vi "Lab Panel V5.24.vi"() -> ()   [LabVIEW 2013] (continued)
                      tunnel: w2146 -> [w2161 _]
                      tunnel: w2145 -> [w2160 _]
                      tunnel: w2144 -> [w2159 _]
                      frame True {
                        n1125 = stacked-sequence {
                          tunnel: w2162 -> [w2166 _]
                          tunnel: w2161 -> [w2164 w2170]
                          tunnel: w2160 -> [_ w2173]
                          tunnel: w2159 -> [w2163 _]
                          frame #0 {
                            n1126 = Build Array(w2164) -> (w2167:string[])
                            n1127 = Build Array(w2166) -> (w2165:dbl[])
                            n1128 = TDMS Write(0:w2163, 5:"TEST PASS", 7:w2167, 9:w2165) -> (15:w2169:errorcluster)  [unwired: 2 in, 3 out]
                            n1129 = local write "data file error"(w2169) -> ()
                          }
                          frame #1 {
                            n1130 = Bundle(cluster=w2173, "STATUS"=w2170) -> (w2171:T4)  [unwired: 2 in]
                            n1131 = local write "RESULT LAB01-2"(TRUE) -> ()
                            n1132 = local write "DISP LAB01-2"(w2171) -> ()
                          }
                        }
                      }
                      frame False {
                      }
                    }
                  }
                }
              }
              frame #2 {
                # "LAB02-1"
                n1133 = Less?(x=w2174, y=2) -> (x < y?=w2177:bool)
                n1134 = local read "DISP LAB02-1"() -> (w2179:T4)
                n1135 = Unbundle(w2179) -> ("STATUS"=w2180:string)  [unwired: 2 out]
                n1136 = Equal?(x=w2180, y="RUN") -> (x = y?=w2176:bool)
                n1137 = And(x=w2176, y=w2177) -> (x .and. y?=w2175:bool)
                n1138 = case shown="True" w2175 {
                  tunnel: w2179 -> [_ w2185]
                  tunnel: w2174 -> [_ w2189]
                  frame False {
                  }
                  frame True {
                    n1139 = local read "SET LAB02-1"() -> (w2191:T5)
                    n1140 = local read "TDMS LAB02-1"() -> (w2184:refnum<k34>)
                    n1141 = Unbundle(w2185) -> ("CYCLE"=w2190:dbl)  [unwired: 2 out]
                    n1142 = Unbundle(w2191) -> ("CYCLES"=w2182:dbl, "T-RISE mins"=w2188:dbl)  [unwired: 3 out]
                    n1143 = case shown="\"T-RISE TEST\"" w2189 {
                      tunnel: w2188 -> [_ _ w2198]
                      tunnel: [w2193 w2195 w2198] -> w2187
                      tunnel: w2182 -> [w2193 w2195 _]
                      tunnel: ["CHART PASS" "CYCLE PASS" "T-RISE PASS"] -> w2186
                      frame "CHART TEST", Default {
                      }
                      frame "CYCLE TEST" {
                      }
                      frame "T-RISE TEST" {
                      }
                    }
                    n1144 = Increment(x=w2182) -> (x+1=w2183:dbl)
                    n1145 = Greater Or Equal?(x=w2190, y=w2183) -> (x >= y?=w2192:bool)
                    n1146 = case shown="True" w2192 {
                      tunnel: w2187 -> [w2202 _]
                      tunnel: w2186 -> [w2201 _]
                      tunnel: w2185 -> [w2200 _]
                      tunnel: w2184 -> [w2199 _]
                      frame True {
                        n1147 = stacked-sequence {
                          tunnel: w2202 -> [w2206 _]
                          tunnel: w2201 -> [w2204 w2210]
                          tunnel: w2200 -> [_ w2213]
                          tunnel: w2199 -> [w2203 _]
                          frame #0 {
                            n1148 = Build Array(w2204) -> (w2207:string[])
                            n1149 = Build Array(w2206) -> (w2205:dbl[])
                            n1150 = TDMS Write(0:w2203, 5:"TEST PASS", 7:w2207, 9:w2205) -> (15:w2209:errorcluster)  [unwired: 2 in, 3 out]
                            n1151 = local write "data file error"(w2209) -> ()
                          }
                          frame #1 {
                            n1152 = Bundle(cluster=w2213, "STATUS"=w2210) -> (w2211:T4)  [unwired: 2 in]
                            n1153 = local write "RESULT LAB02-1"(TRUE) -> ()
                            n1154 = local write "DISP LAB02-1"(w2211) -> ()
                          }
                        }
                      }
                      frame False {
                      }
                    }
                  }
                }
              }
              frame #3 {
                # "LAB02-2"
                n1155 = Less?(x=w2214, y=2) -> (x < y?=w2217:bool)
                n1156 = local read "DISP LAB02-2"() -> (w2219:T4)
                n1157 = Unbundle(w2219) -> ("STATUS"=w2220:string)  [unwired: 2 out]
                n1158 = Equal?(x=w2220, y="RUN") -> (x = y?=w2216:bool)
                n1159 = And(x=w2216, y=w2217) -> (x .and. y?=w2215:bool)
                n1160 = case shown="True" w2215 {
                  tunnel: w2219 -> [_ w2225]
                  tunnel: w2214 -> [_ w2229]
                  frame False {
                  }
                  frame True {
                    n1161 = local read "SET LAB02-2"() -> (w2231:T5)
                    n1162 = local read "TDMS LAB02-2"() -> (w2224:refnum<k34>)
                    n1163 = Unbundle(w2225) -> ("CYCLE"=w2230:dbl)  [unwired: 2 out]
                    n1164 = Unbundle(w2231) -> ("CYCLES"=w2222:dbl, "T-RISE mins"=w2228:dbl)  [unwired: 3 out]
                    n1165 = case shown="\"T-RISE TEST\"" w2229 {
                      tunnel: w2228 -> [_ _ w2238]
                      tunnel: [w2233 w2235 w2238] -> w2227
                      tunnel: w2222 -> [w2233 w2235 _]
                      tunnel: ["CHART PASS" "CYCLE PASS" "T-RISE PASS"] -> w2226
                      frame "CHART TEST", Default {
                      }
                      frame "CYCLE TEST" {
                      }
                      frame "T-RISE TEST" {
                      }
                    }
                    n1166 = Increment(x=w2222) -> (x+1=w2223:dbl)
                    n1167 = Greater Or Equal?(x=w2230, y=w2223) -> (x >= y?=w2232:bool)
                    n1168 = case shown="True" w2232 {
                      tunnel: w2227 -> [w2242 _]
                      tunnel: w2226 -> [w2241 _]
                      tunnel: w2225 -> [w2240 _]
                      tunnel: w2224 -> [w2239 _]
                      frame True {
                        n1169 = stacked-sequence {
                          tunnel: w2242 -> [w2246 _]
                          tunnel: w2241 -> [w2244 w2250]
                          tunnel: w2240 -> [_ w2253]
                          tunnel: w2239 -> [w2243 _]
                          frame #0 {
                            n1170 = Build Array(w2244) -> (w2247:string[])
                            n1171 = Build Array(w2246) -> (w2245:dbl[])
                            n1172 = TDMS Write(0:w2243, 5:"TEST PASS", 7:w2247, 9:w2245) -> (15:w2249:errorcluster)  [unwired: 2 in, 3 out]
                            n1173 = local write "data file error"(w2249) -> ()
                          }
                          frame #1 {
                            n1174 = Bundle(cluster=w2253, "STATUS"=w2250) -> (w2251:T4)  [unwired: 2 in]
                            n1175 = local write "RESULT LAB02-2"(TRUE) -> ()
                            n1176 = local write "DISP LAB02-2"(w2251) -> ()
                          }
                        }
                      }
                      frame False {
                      }
                    }
                  }
                }
              }
              frame #4 {
                # "LAB03-1"
                n1177 = Less?(x=w2254, y=2) -> (x < y?=w2257:bool)
                n1178 = local read "DISP LAB03-1"() -> (w2259:T4)
                n1179 = Unbundle(w2259) -> ("STATUS"=w2260:string)  [unwired: 2 out]
                n1180 = Equal?(x=w2260, y="RUN") -> (x = y?=w2256:bool)
                n1181 = And(x=w2256, y=w2257) -> (x .and. y?=w2255:bool)
                n1182 = case shown="True" w2255 {
                  tunnel: w2259 -> [_ w2265]
                  tunnel: w2254 -> [_ w2269]
                  frame False {
                  }
                  frame True {
                    n1183 = local read "SET LAB03-1"() -> (w2271:T5)
                    n1184 = local read "TDMS LAB03-1"() -> (w2264:refnum<k34>)
                    n1185 = Unbundle(w2265) -> ("CYCLE"=w2270:dbl)  [unwired: 2 out]
                    n1186 = Unbundle(w2271) -> ("CYCLES"=w2262:dbl, "T-RISE mins"=w2268:dbl)  [unwired: 3 out]
                    n1187 = case shown="\"T-RISE TEST\"" w2269 {
                      tunnel: w2268 -> [_ _ w2278]
                      tunnel: [w2273 w2275 w2278] -> w2267
                      tunnel: w2262 -> [w2273 w2275 _]
                      tunnel: ["CHART PASS" "CYCLE PASS" "T-RISE PASS"] -> w2266
                      frame "CHART TEST", Default {
                      }
                      frame "CYCLE TEST" {
                      }
                      frame "T-RISE TEST" {
                      }
                    }
                    n1188 = Increment(x=w2262) -> (x+1=w2263:dbl)
                    n1189 = Greater Or Equal?(x=w2270, y=w2263) -> (x >= y?=w2272:bool)
                    n1190 = case shown="True" w2272 {
                      tunnel: w2267 -> [w2282 _]
                      tunnel: w2266 -> [w2281 _]
                      tunnel: w2265 -> [w2280 _]
                      tunnel: w2264 -> [w2279 _]
                      frame True {
                        n1191 = stacked-sequence {
                          tunnel: w2282 -> [w2286 _]
                          tunnel: w2281 -> [w2284 w2290]
                          tunnel: w2280 -> [_ w2293]
                          tunnel: w2279 -> [w2283 _]
                          frame #0 {
                            n1192 = Build Array(w2284) -> (w2287:string[])
                            n1193 = Build Array(w2286) -> (w2285:dbl[])
                            n1194 = TDMS Write(0:w2283, 5:"TEST PASS", 7:w2287, 9:w2285) -> (15:w2289:errorcluster)  [unwired: 2 in, 3 out]
                            n1195 = local write "data file error"(w2289) -> ()
                          }
                          frame #1 {
                            n1196 = Bundle(cluster=w2293, "STATUS"=w2290) -> (w2291:T4)  [unwired: 2 in]
                            n1197 = local write "RESULT LAB03-1"(TRUE) -> ()
                            n1198 = local write "DISP LAB03-1"(w2291) -> ()
                          }
                        }
                      }
                      frame False {
                      }
                    }
                  }
                }
              }
              frame #5 {
                # "LAB03-2"
                n1199 = Less?(x=w2294, y=2) -> (x < y?=w2297:bool)
                n1200 = local read "DISP LAB03-2"() -> (w2299:T4)
                n1201 = Unbundle(w2299) -> ("STATUS"=w2300:string)  [unwired: 2 out]
                n1202 = Equal?(x=w2300, y="RUN") -> (x = y?=w2296:bool)
                n1203 = And(x=w2296, y=w2297) -> (x .and. y?=w2295:bool)
                n1204 = case shown="True" w2295 {
                  tunnel: w2299 -> [_ w2305]
                  tunnel: w2294 -> [_ w2309]
                  frame False {
                  }
                  frame True {
                    n1205 = local read "SET LAB03-2"() -> (w2311:T5)
                    n1206 = local read "TDMS LAB03-2"() -> (w2304:refnum<k34>)
                    n1207 = Unbundle(w2305) -> ("CYCLE"=w2310:dbl)  [unwired: 2 out]
                    n1208 = Unbundle(w2311) -> ("CYCLES"=w2302:dbl, "T-RISE mins"=w2308:dbl)  [unwired: 3 out]
                    n1209 = case shown="\"T-RISE TEST\"" w2309 {
                      tunnel: w2308 -> [_ _ w2318]
                      tunnel: [w2313 w2315 w2318] -> w2307
                      tunnel: w2302 -> [w2313 w2315 _]
                      tunnel: ["CHART PASS" "CYCLE PASS" "T-RISE PASS"] -> w2306
                      frame "CHART TEST", Default {
                      }
                      frame "CYCLE TEST" {
                      }
                      frame "T-RISE TEST" {
                      }
                    }
                    n1210 = Increment(x=w2302) -> (x+1=w2303:dbl)
                    n1211 = Greater Or Equal?(x=w2310, y=w2303) -> (x >= y?=w2312:bool)
                    n1212 = case shown="True" w2312 {
                      tunnel: w2307 -> [w2322 _]
                      tunnel: w2306 -> [w2321 _]
                      tunnel: w2305 -> [w2320 _]
                      tunnel: w2304 -> [w2319 _]
                      frame True {
                        n1213 = stacked-sequence {
                          tunnel: w2322 -> [w2326 _]
                          tunnel: w2321 -> [w2324 w2330]
                          tunnel: w2320 -> [_ w2333]
                          tunnel: w2319 -> [w2323 _]
                          frame #0 {
                            n1214 = Build Array(w2324) -> (w2327:string[])
                            n1215 = Build Array(w2326) -> (w2325:dbl[])
                            n1216 = TDMS Write(0:w2323, 5:"TEST PASS", 7:w2327, 9:w2325) -> (15:w2329:errorcluster)  [unwired: 2 in, 3 out]
                            n1217 = local write "data file error"(w2329) -> ()
                          }
                          frame #1 {
                            n1218 = Bundle(cluster=w2333, "STATUS"=w2330) -> (w2331:T4)  [unwired: 2 in]
                            n1219 = local write "RESULT LAB03-2"(TRUE) -> ()
                            n1220 = local write "DISP LAB03-2"(w2331) -> ()
                          }
                        }
                      }
                      frame False {
                      }
                    }
                  }
                }
              }
              frame #6 {
                # "LAB04-1"
                n1221 = Less?(x=w2334, y=2) -> (x < y?=w2337:bool)
                n1222 = local read "DISP LAB04-1"() -> (w2339:T4)
                n1223 = Unbundle(w2339) -> ("STATUS"=w2340:string)  [unwired: 2 out]
                n1224 = Equal?(x=w2340, y="RUN") -> (x = y?=w2336:bool)
                n1225 = And(x=w2336, y=w2337) -> (x .and. y?=w2335:bool)
                n1226 = case shown="True" w2335 {
                  tunnel: w2339 -> [_ w2345]
                  tunnel: w2334 -> [_ w2349]
                  frame False {
                  }
                  frame True {
                    n1227 = local read "SET LAB04-1"() -> (w2351:T5)
                    n1228 = local read "TDMS LAB04-1"() -> (w2344:refnum<k34>)
                    n1229 = Unbundle(w2345) -> ("CYCLE"=w2350:dbl)  [unwired: 2 out]
                    n1230 = Unbundle(w2351) -> ("CYCLES"=w2342:dbl, "T-RISE mins"=w2348:dbl)  [unwired: 3 out]
                    n1231 = case shown="\"T-RISE TEST\"" w2349 {
                      tunnel: w2348 -> [_ _ w2358]
                      tunnel: [w2353 w2355 w2358] -> w2347
                      tunnel: w2342 -> [w2353 w2355 _]
                      tunnel: ["CHART PASS" "CYCLE PASS" "T-RISE PASS"] -> w2346
                      frame "CHART TEST", Default {
                      }
                      frame "CYCLE TEST" {
                      }
                      frame "T-RISE TEST" {
                      }
                    }
                    n1232 = Increment(x=w2342) -> (x+1=w2343:dbl)
                    n1233 = Greater Or Equal?(x=w2350, y=w2343) -> (x >= y?=w2352:bool)
                    n1234 = case shown="True" w2352 {
                      tunnel: w2347 -> [w2362 _]
                      tunnel: w2346 -> [w2361 _]
                      tunnel: w2345 -> [w2360 _]
                      tunnel: w2344 -> [w2359 _]
                      frame True {
                        n1235 = stacked-sequence {
                          tunnel: w2362 -> [w2366 _]
                          tunnel: w2361 -> [w2364 w2370]
                          tunnel: w2360 -> [_ w2373]
                          tunnel: w2359 -> [w2363 _]
                          frame #0 {
                            n1236 = Build Array(w2364) -> (w2367:string[])
                            n1237 = Build Array(w2366) -> (w2365:dbl[])
                            n1238 = TDMS Write(0:w2363, 5:"TEST PASS", 7:w2367, 9:w2365) -> (15:w2369:errorcluster)  [unwired: 2 in, 3 out]
                            n1239 = local write "data file error"(w2369) -> ()
                          }
                          frame #1 {
                            n1240 = Bundle(cluster=w2373, "STATUS"=w2370) -> (w2371:T4)  [unwired: 2 in]
                            n1241 = local write "RESULT LAB04-1"(TRUE) -> ()
                            n1242 = local write "DISP LAB04-1"(w2371) -> ()
                          }
                        }
                      }
                      frame False {
                      }
                    }
                  }
                }
              }
              frame #7 {
                # "LAB04-2"
                n1243 = Less?(x=w2374, y=2) -> (x < y?=w2377:bool)
                n1244 = local read "DISP LAB04-2"() -> (w2379:T4)
                n1245 = Unbundle(w2379) -> ("STATUS"=w2380:string)  [unwired: 2 out]
                n1246 = Equal?(x=w2380, y="RUN") -> (x = y?=w2376:bool)
                n1247 = And(x=w2376, y=w2377) -> (x .and. y?=w2375:bool)
                n1248 = case shown="True" w2375 {
                  tunnel: w2379 -> [_ w2385]
                  tunnel: w2374 -> [_ w2389]
                  frame False {
                  }
                  frame True {
                    n1249 = local read "SET LAB04-2"() -> (w2391:T5)
                    n1250 = local read "TDMS LAB04-2"() -> (w2384:refnum<k34>)
                    n1251 = Unbundle(w2385) -> ("CYCLE"=w2390:dbl)  [unwired: 2 out]
                    n1252 = Unbundle(w2391) -> ("CYCLES"=w2382:dbl, "T-RISE mins"=w2388:dbl)  [unwired: 3 out]
                    n1253 = case shown="\"T-RISE TEST\"" w2389 {
                      tunnel: w2388 -> [_ _ w2398]
                      tunnel: [w2393 w2395 w2398] -> w2387
                      tunnel: w2382 -> [w2393 w2395 _]
                      tunnel: ["CHART PASS" "CYCLE PASS" "T-RISE PASS"] -> w2386
                      frame "CHART TEST", Default {
                      }
                      frame "CYCLE TEST" {
                      }
                      frame "T-RISE TEST" {
                      }
                    }
                    n1254 = Increment(x=w2382) -> (x+1=w2383:dbl)
                    n1255 = Greater Or Equal?(x=w2390, y=w2383) -> (x >= y?=w2392:bool)
                    n1256 = case shown="True" w2392 {
                      tunnel: w2387 -> [w2402 _]
                      tunnel: w2386 -> [w2401 _]
                      tunnel: w2385 -> [w2400 _]
                      tunnel: w2384 -> [w2399 _]
                      frame True {
                        n1257 = stacked-sequence {
                          tunnel: w2402 -> [w2406 _]
                          tunnel: w2401 -> [w2404 w2410]
                          tunnel: w2400 -> [_ w2413]
                          tunnel: w2399 -> [w2403 _]
                          frame #0 {
                            n1258 = Build Array(w2404) -> (w2407:string[])
                            n1259 = Build Array(w2406) -> (w2405:dbl[])
                            n1260 = TDMS Write(0:w2403, 5:"TEST PASS", 7:w2407, 9:w2405) -> (15:w2409:errorcluster)  [unwired: 2 in, 3 out]
                            n1261 = local write "data file error"(w2409) -> ()
                          }
                          frame #1 {
                            n1262 = Bundle(cluster=w2413, "STATUS"=w2410) -> (w2411:T4)  [unwired: 2 in]
                            n1263 = local write "RESULT LAB04-2"(TRUE) -> ()
                            n1264 = local write "DISP LAB04-2"(w2411) -> ()
                          }
                        }
                      }
                      frame False {
                      }
                    }
                  }
                }
              }
              frame #8 {
                # "LAB05-1"
                n1265 = Less?(x=w2414, y=2) -> (x < y?=w2417:bool)
                n1266 = local read "DISP LAB05-1"() -> (w2419:T4)
                n1267 = Unbundle(w2419) -> ("STATUS"=w2420:string)  [unwired: 2 out]
                n1268 = Equal?(x=w2420, y="RUN") -> (x = y?=w2416:bool)
                n1269 = And(x=w2416, y=w2417) -> (x .and. y?=w2415:bool)
                n1270 = case shown="True" w2415 {
                  tunnel: w2419 -> [_ w2425]
                  tunnel: w2414 -> [_ w2429]
                  frame False {
                  }
                  frame True {
                    n1271 = local read "SET LAB05-1"() -> (w2431:T5)
                    n1272 = local read "TDMS LAB05-1"() -> (w2424:refnum<k34>)
                    n1273 = Unbundle(w2425) -> ("CYCLE"=w2430:dbl)  [unwired: 2 out]
                    n1274 = Unbundle(w2431) -> ("CYCLES"=w2422:dbl, "T-RISE mins"=w2428:dbl)  [unwired: 3 out]
                    n1275 = case shown="\"T-RISE TEST\"" w2429 {
                      tunnel: w2428 -> [_ _ w2438]
                      tunnel: [w2433 w2435 w2438] -> w2427
                      tunnel: w2422 -> [w2433 w2435 _]
                      tunnel: ["CHART PASS" "CYCLE PASS" "T-RISE PASS"] -> w2426
                      frame "CHART TEST", Default {
                      }
                      frame "CYCLE TEST" {
                      }
                      frame "T-RISE TEST" {
                      }
                    }
                    n1276 = Increment(x=w2422) -> (x+1=w2423:dbl)
                    n1277 = Greater Or Equal?(x=w2430, y=w2423) -> (x >= y?=w2432:bool)
                    n1278 = case shown="True" w2432 {
                      tunnel: w2427 -> [w2442 _]
                      tunnel: w2426 -> [w2441 _]
                      tunnel: w2425 -> [w2440 _]
                      tunnel: w2424 -> [w2439 _]
                      frame True {
                        n1279 = stacked-sequence {
                          tunnel: w2442 -> [w2446 _]
                          tunnel: w2441 -> [w2444 w2450]
                          tunnel: w2440 -> [_ w2453]
                          tunnel: w2439 -> [w2443 _]
                          frame #0 {
                            n1280 = Build Array(w2444) -> (w2447:string[])
                            n1281 = Build Array(w2446) -> (w2445:dbl[])
                            n1282 = TDMS Write(0:w2443, 5:"TEST PASS", 7:w2447, 9:w2445) -> (15:w2449:errorcluster)  [unwired: 2 in, 3 out]
                            n1283 = local write "data file error"(w2449) -> ()
                          }
                          frame #1 {
                            n1284 = Bundle(cluster=w2453, "STATUS"=w2450) -> (w2451:T4)  [unwired: 2 in]
                            n1285 = local write "RESULT LAB05-1"(TRUE) -> ()
                            n1286 = local write "DISP LAB05-1"(w2451) -> ()
                          }
                        }
                      }
                      frame False {
                      }
                    }
                  }
                }
              }
              frame #9 {
                # "LAB05-2"
                n1287 = Less?(x=w2454, y=2) -> (x < y?=w2457:bool)
                n1288 = local read "DISP LAB05-2"() -> (w2459:T4)
                n1289 = Unbundle(w2459) -> ("STATUS"=w2460:string)  [unwired: 2 out]
                n1290 = Equal?(x=w2460, y="RUN") -> (x = y?=w2456:bool)
                n1291 = And(x=w2456, y=w2457) -> (x .and. y?=w2455:bool)
                n1292 = case shown="True" w2455 {
                  tunnel: w2459 -> [_ w2465]
                  tunnel: w2454 -> [_ w2469]
                  frame False {
                  }
                  frame True {
                    n1293 = local read "SET LAB05-2"() -> (w2471:T5)
                    n1294 = local read "TDMS LAB05-2"() -> (w2464:refnum<k34>)
                    n1295 = Unbundle(w2465) -> ("CYCLE"=w2470:dbl)  [unwired: 2 out]
                    n1296 = Unbundle(w2471) -> ("CYCLES"=w2462:dbl, "T-RISE mins"=w2468:dbl)  [unwired: 3 out]
                    n1297 = case shown="\"T-RISE TEST\"" w2469 {
                      tunnel: w2468 -> [_ _ w2478]
                      tunnel: [w2473 w2475 w2478] -> w2467
                      tunnel: w2462 -> [w2473 w2475 _]
                      tunnel: ["CHART PASS" "CYCLE PASS" "T-RISE PASS"] -> w2466
                      frame "CHART TEST", Default {
                      }
                      frame "CYCLE TEST" {
                      }
                      frame "T-RISE TEST" {
                      }
                    }
                    n1298 = Increment(x=w2462) -> (x+1=w2463:dbl)
                    n1299 = Greater Or Equal?(x=w2470, y=w2463) -> (x >= y?=w2472:bool)
                    n1300 = case shown="True" w2472 {
                      tunnel: w2467 -> [w2482 _]
                      tunnel: w2466 -> [w2481 _]
                      tunnel: w2465 -> [w2480 _]
                      tunnel: w2464 -> [w2479 _]
                      frame True {
                        n1301 = stacked-sequence {
                          tunnel: w2482 -> [w2486 _]
                          tunnel: w2481 -> [w2484 w2490]
                          tunnel: w2480 -> [_ w2493]
                          tunnel: w2479 -> [w2483 _]
                          frame #0 {
                            n1302 = Build Array(w2484) -> (w2487:string[])
                            n1303 = Build Array(w2486) -> (w2485:dbl[])
                            n1304 = TDMS Write(0:w2483, 5:"TEST PASS", 7:w2487, 9:w2485) -> (15:w2489:errorcluster)  [unwired: 2 in, 3 out]
                            n1305 = local write "data file error"(w2489) -> ()
                          }
                          frame #1 {
                            n1306 = Bundle(cluster=w2493, "STATUS"=w2490) -> (w2491:T4)  [unwired: 2 in]
                            n1307 = local write "RESULT LAB05-2"(TRUE) -> ()
                            n1308 = local write "DISP LAB05-2"(w2491) -> ()
                          }
                        }
                      }
                      frame False {
                      }
                    }
                  }
                }
              }
            }
          }
          frame #5 {
            # "check if test cycles reached for temperature rise test"
            n1309 = stacked-sequence {
              tunnel: w2523 -> [_ _ _ _ _ _ _ _ _ _]
              tunnel: w2522 -> [_ _ _ _ _ _ _ _ _ _]
              tunnel: w2521 -> [_ _ _ _ _ _ _ _ _ _]
              tunnel: w2520 -> [_ _ _ _ _ _ _ _ _ _]
              tunnel: w2519 -> [_ _ _ _ _ _ _ _ _ _]
              tunnel: w2518 -> [_ _ _ _ _ _ _ _ _ _]
              tunnel: w2517 -> [_ _ _ _ _ _ _ _ _ _]
              tunnel: w2516 -> [_ _ _ _ _ _ _ _ _ _]
              tunnel: w2515 -> [_ _ _ _ _ _ _ _ _ _]
              tunnel: w2514 -> [_ _ _ _ _ _ _ _ _ _]
              tunnel: w2513 -> [w2529 _ _ _ _ _ _ _ _ _]
              tunnel: w2503 -> [w2524 _ _ _ _ _ _ _ _ _]
              tunnel: w2512 -> [_ w2555 _ _ _ _ _ _ _ _]
              tunnel: w2511 -> [_ _ w2585 _ _ _ _ _ _ _]
              tunnel: w2510 -> [_ _ _ w2615 _ _ _ _ _ _]
              tunnel: w2509 -> [_ _ _ _ w2645 _ _ _ _ _]
              tunnel: w2508 -> [_ _ _ _ _ w2675 _ _ _ _]
              tunnel: w2507 -> [_ _ _ _ _ _ w2705 _ _ _]
              tunnel: w2506 -> [_ _ _ _ _ _ _ w2735 _ _]
              tunnel: w2505 -> [_ _ _ _ _ _ _ _ w2765 _]
              tunnel: w2504 -> [_ _ _ _ _ _ _ _ _ w2795]
              tunnel: w2502 -> [_ w2554 _ _ _ _ _ _ _ _]
              tunnel: w2501 -> [_ _ w2584 _ _ _ _ _ _ _]
              tunnel: w2500 -> [_ _ _ w2614 _ _ _ _ _ _]
              tunnel: w2499 -> [_ _ _ _ w2644 _ _ _ _ _]
              tunnel: w2498 -> [_ _ _ _ _ w2674 _ _ _ _]
              tunnel: w2497 -> [_ _ _ _ _ _ w2704 _ _ _]
              tunnel: w2496 -> [_ _ _ _ _ _ _ w2734 _ _]
              tunnel: w2495 -> [_ _ _ _ _ _ _ _ w2764 _]
              tunnel: w2494 -> [_ _ _ _ _ _ _ _ _ w2794]
              frame #0 {
                # "LAB01-1"
                n1310 = Equal?(x=w2529, y=2) -> (x = y?=w2527:bool)
                n1311 = local read "DISP LAB01-1"() -> (w2530:T4)
                n1312 = Unbundle(w2530) -> ("STATUS"=w2531:string)  [unwired: 2 out]
                n1313 = Equal?(x=w2531, y="RUN") -> (x = y?=w2526:bool)
                n1314 = And(x=w2526, y=w2527) -> (x .and. y?=w2525:bool)
                n1315 = case shown="True" w2525 {
                  tunnel: w2530 -> [_ w2534]
                  tunnel: w2524 -> [_ w2537]
                  frame False {
                  }
                  frame True {
                    n1316 = local read "SET LAB01-1"() -> (w2536:T5)
                    n1317 = local read "TDMS LAB01-1"() -> (w2533:refnum<k34>)
                    n1318 = Unbundle(w2534) -> ("CYCLE"=w2538:dbl)  [unwired: 2 out]
                    n1319 = Unbundle(w2536) -> ("T-RISE mins"=w2535:dbl)  [unwired: 4 out]
                    n1320 = Greater Or Equal?(x=w2538, y=w2537) -> (x >= y?=w2539:bool)
                    n1321 = case shown="True" w2539 {
                      tunnel: w2535 -> [w2542 _]
                      tunnel: w2534 -> [w2541 _]
                      tunnel: w2533 -> [w2540 _]
                      frame True {
                        n1322 = stacked-sequence {
                          tunnel: w2542 -> [w2545 _]
                          tunnel: w2541 -> [_ w2550]
                          tunnel: w2540 -> [w2543 _]
                          frame #0 {
                            n1323 = Build Array("T-RISE") -> (w2547:string[])
                            n1324 = Build Array(w2545) -> (w2546:dbl[])
                            n1325 = TDMS Write(0:w2543, 5:"TEST PASS", 7:w2547, 9:w2546) -> (15:w2549:errorcluster)  [unwired: 2 in, 3 out]
                            n1326 = local write "data file error"(w2549) -> ()
                          }
                          frame #1 {
                            n1327 = Bundle(cluster=w2550, "STATUS"="T-RISE PASS") -> (w2552:T4)  [unwired: 2 in]
                            n1328 = local write "RESULT LAB01-1"(TRUE) -> ()
                            n1329 = local write "DISP LAB01-1"(w2552) -> ()
                          }
                        }
                      }
                      frame False {
                      }
                    }
                  }
                }
              }
              frame #1 {
                # "LAB01-2"
                n1330 = Equal?(x=w2555, y=2) -> (x = y?=w2558:bool)
                n1331 = local read "DISP LAB01-2"() -> (w2560:T4)
                n1332 = Unbundle(w2560) -> ("STATUS"=w2561:string)  [unwired: 2 out]
                n1333 = Equal?(x=w2561, y="RUN") -> (x = y?=w2557:bool)
                n1334 = And(x=w2557, y=w2558) -> (x .and. y?=w2556:bool)
                n1335 = case shown="True" w2556 {
                  tunnel: w2560 -> [_ w2564]
                  tunnel: w2554 -> [_ w2567]
                  frame False {
                  }
                  frame True {
                    n1336 = local read "SET LAB01-2"() -> (w2566:T5)
                    n1337 = local read "TDMS LAB01-2"() -> (w2563:refnum<k34>)
                    n1338 = Unbundle(w2564) -> ("CYCLE"=w2568:dbl)  [unwired: 2 out]
                    n1339 = Unbundle(w2566) -> ("T-RISE mins"=w2565:dbl)  [unwired: 4 out]
                    n1340 = Greater Or Equal?(x=w2568, y=w2567) -> (x >= y?=w2569:bool)
                    n1341 = case shown="True" w2569 {
                      tunnel: w2565 -> [w2572 _]
                      tunnel: w2564 -> [w2571 _]
                      tunnel: w2563 -> [w2570 _]
                      frame True {
                        n1342 = stacked-sequence {
                          tunnel: w2572 -> [w2575 _]
                          tunnel: w2571 -> [_ w2580]
                          tunnel: w2570 -> [w2573 _]
                          frame #0 {
                            n1343 = Build Array("T-RISE") -> (w2577:string[])
                            n1344 = Build Array(w2575) -> (w2576:dbl[])
                            n1345 = TDMS Write(0:w2573, 5:"TEST PASS", 7:w2577, 9:w2576) -> (15:w2579:errorcluster)  [unwired: 2 in, 3 out]
                            n1346 = local write "data file error"(w2579) -> ()
                          }
                          frame #1 {
                            n1347 = Bundle(cluster=w2580, "STATUS"="T-RISE PASS") -> (w2582:T4)  [unwired: 2 in]
                            n1348 = local write "RESULT LAB01-2"(TRUE) -> ()
                            n1349 = local write "DISP LAB01-2"(w2582) -> ()
                          }
                        }
                      }
                      frame False {
                      }
                    }
                  }
                }
              }
              frame #2 {
                # "LAB02-1"
                n1350 = Equal?(x=w2585, y=2) -> (x = y?=w2588:bool)
                n1351 = local read "DISP LAB02-1"() -> (w2590:T4)
                n1352 = Unbundle(w2590) -> ("STATUS"=w2591:string)  [unwired: 2 out]
                n1353 = Equal?(x=w2591, y="RUN") -> (x = y?=w2587:bool)
                n1354 = And(x=w2587, y=w2588) -> (x .and. y?=w2586:bool)
                n1355 = case shown="True" w2586 {
                  tunnel: w2590 -> [_ w2594]
                  tunnel: w2584 -> [_ w2597]
                  frame False {
                  }
                  frame True {
                    n1356 = local read "SET LAB02-1"() -> (w2596:T5)
                    n1357 = local read "TDMS LAB02-1"() -> (w2593:refnum<k34>)
                    n1358 = Unbundle(w2594) -> ("CYCLE"=w2598:dbl)  [unwired: 2 out]
                    n1359 = Unbundle(w2596) -> ("T-RISE mins"=w2595:dbl)  [unwired: 4 out]
                    n1360 = Greater Or Equal?(x=w2598, y=w2597) -> (x >= y?=w2599:bool)
                    n1361 = case shown="True" w2599 {
                      tunnel: w2595 -> [w2602 _]
                      tunnel: w2594 -> [w2601 _]
                      tunnel: w2593 -> [w2600 _]
                      frame True {
                        n1362 = stacked-sequence {
                          tunnel: w2602 -> [w2605 _]
                          tunnel: w2601 -> [_ w2610]
                          tunnel: w2600 -> [w2603 _]
                          frame #0 {
                            n1363 = Build Array("T-RISE") -> (w2607:string[])
                            n1364 = Build Array(w2605) -> (w2606:dbl[])
                            n1365 = TDMS Write(0:w2603, 5:"TEST PASS", 7:w2607, 9:w2606) -> (15:w2609:errorcluster)  [unwired: 2 in, 3 out]
                            n1366 = local write "data file error"(w2609) -> ()
                          }
                          frame #1 {
                            n1367 = Bundle(cluster=w2610, "STATUS"="T-RISE PASS") -> (w2612:T4)  [unwired: 2 in]
                            n1368 = local write "RESULT LAB02-1"(TRUE) -> ()
                            n1369 = local write "DISP LAB02-1"(w2612) -> ()
                          }
                        }
                      }
                      frame False {
                      }
                    }
                  }
                }
              }
              frame #3 {
                # "LAB02-2"
                n1370 = Equal?(x=w2615, y=2) -> (x = y?=w2618:bool)
                n1371 = local read "DISP LAB02-2"() -> (w2620:T4)
                n1372 = Unbundle(w2620) -> ("STATUS"=w2621:string)  [unwired: 2 out]
                n1373 = Equal?(x=w2621, y="RUN") -> (x = y?=w2617:bool)
                n1374 = And(x=w2617, y=w2618) -> (x .and. y?=w2616:bool)
                n1375 = case shown="True" w2616 {
                  tunnel: w2620 -> [_ w2624]
                  tunnel: w2614 -> [_ w2627]
                  frame False {
                  }
                  frame True {
                    n1376 = local read "SET LAB02-2"() -> (w2626:T5)
                    n1377 = local read "TDMS LAB02-2"() -> (w2623:refnum<k34>)
                    n1378 = Unbundle(w2624) -> ("CYCLE"=w2628:dbl)  [unwired: 2 out]
                    n1379 = Unbundle(w2626) -> ("T-RISE mins"=w2625:dbl)  [unwired: 4 out]
                    n1380 = Greater Or Equal?(x=w2628, y=w2627) -> (x >= y?=w2629:bool)
                    n1381 = case shown="True" w2629 {
                      tunnel: w2625 -> [w2632 _]
                      tunnel: w2624 -> [w2631 _]
                      tunnel: w2623 -> [w2630 _]
                      frame True {
                        n1382 = stacked-sequence {
                          tunnel: w2632 -> [w2635 _]
                          tunnel: w2631 -> [_ w2640]
                          tunnel: w2630 -> [w2633 _]
                          frame #0 {
                            n1383 = Build Array("T-RISE") -> (w2637:string[])
                            n1384 = Build Array(w2635) -> (w2636:dbl[])
                            n1385 = TDMS Write(0:w2633, 5:"TEST PASS", 7:w2637, 9:w2636) -> (15:w2639:errorcluster)  [unwired: 2 in, 3 out]
                            n1386 = local write "data file error"(w2639) -> ()
                          }
                          frame #1 {
                            n1387 = Bundle(cluster=w2640, "STATUS"="T-RISE PASS") -> (w2642:T4)  [unwired: 2 in]
                            n1388 = local write "RESULT LAB02-2"(TRUE) -> ()
                            n1389 = local write "DISP LAB02-2"(w2642) -> ()
                          }
                        }
                      }
                      frame False {
                      }
                    }
                  }
                }
              }
              frame #4 {
                # "LAB03-1"
                n1390 = Equal?(x=w2645, y=2) -> (x = y?=w2648:bool)
                n1391 = local read "DISP LAB03-1"() -> (w2650:T4)
                n1392 = Unbundle(w2650) -> ("STATUS"=w2651:string)  [unwired: 2 out]
                n1393 = Equal?(x=w2651, y="RUN") -> (x = y?=w2647:bool)
                n1394 = And(x=w2647, y=w2648) -> (x .and. y?=w2646:bool)
                n1395 = case shown="True" w2646 {
                  tunnel: w2650 -> [_ w2654]
                  tunnel: w2644 -> [_ w2657]
                  frame False {
                  }
                  frame True {
                    n1396 = local read "SET LAB03-1"() -> (w2656:T5)
                    n1397 = local read "TDMS LAB03-1"() -> (w2653:refnum<k34>)
                    n1398 = Unbundle(w2654) -> ("CYCLE"=w2658:dbl)  [unwired: 2 out]
                    n1399 = Unbundle(w2656) -> ("T-RISE mins"=w2655:dbl)  [unwired: 4 out]
                    n1400 = Greater Or Equal?(x=w2658, y=w2657) -> (x >= y?=w2659:bool)
                    n1401 = case shown="True" w2659 {
                      tunnel: w2655 -> [w2662 _]
                      tunnel: w2654 -> [w2661 _]
                      tunnel: w2653 -> [w2660 _]
                      frame True {
                        n1402 = stacked-sequence {
                          tunnel: w2662 -> [w2665 _]
                          tunnel: w2661 -> [_ w2670]
                          tunnel: w2660 -> [w2663 _]
                          frame #0 {
                            n1403 = Build Array("T-RISE") -> (w2667:string[])
                            n1404 = Build Array(w2665) -> (w2666:dbl[])
                            n1405 = TDMS Write(0:w2663, 5:"TEST PASS", 7:w2667, 9:w2666) -> (15:w2669:errorcluster)  [unwired: 2 in, 3 out]
                            n1406 = local write "data file error"(w2669) -> ()
                          }
                          frame #1 {
                            n1407 = Bundle(cluster=w2670, "STATUS"="T-RISE PASS") -> (w2672:T4)  [unwired: 2 in]
                            n1408 = local write "RESULT LAB03-1"(TRUE) -> ()
                            n1409 = local write "DISP LAB03-1"(w2672) -> ()
                          }
                        }
                      }
                      frame False {
                      }
                    }
                  }
                }
              }
              frame #5 {
                # "LAB03-2"
                n1410 = Equal?(x=w2675, y=2) -> (x = y?=w2678:bool)
                n1411 = local read "DISP LAB03-2"() -> (w2680:T4)
                n1412 = Unbundle(w2680) -> ("STATUS"=w2681:string)  [unwired: 2 out]
                n1413 = Equal?(x=w2681, y="RUN") -> (x = y?=w2677:bool)
                n1414 = And(x=w2677, y=w2678) -> (x .and. y?=w2676:bool)
                n1415 = case shown="True" w2676 {
                  tunnel: w2680 -> [_ w2684]
                  tunnel: w2674 -> [_ w2687]
                  frame False {
                  }
                  frame True {
                    n1416 = local read "SET LAB03-2"() -> (w2686:T5)
                    n1417 = local read "TDMS LAB03-2"() -> (w2683:refnum<k34>)
                    n1418 = Unbundle(w2684) -> ("CYCLE"=w2688:dbl)  [unwired: 2 out]
                    n1419 = Unbundle(w2686) -> ("T-RISE mins"=w2685:dbl)  [unwired: 4 out]
                    n1420 = Greater Or Equal?(x=w2688, y=w2687) -> (x >= y?=w2689:bool)
                    n1421 = case shown="True" w2689 {
                      tunnel: w2685 -> [w2692 _]
                      tunnel: w2684 -> [w2691 _]
                      tunnel: w2683 -> [w2690 _]
                      frame True {
                        n1422 = stacked-sequence {
                          tunnel: w2692 -> [w2695 _]
                          tunnel: w2691 -> [_ w2700]
                          tunnel: w2690 -> [w2693 _]
                          frame #0 {
                            n1423 = Build Array("T-RISE") -> (w2697:string[])
                            n1424 = Build Array(w2695) -> (w2696:dbl[])
                            n1425 = TDMS Write(0:w2693, 5:"TEST PASS", 7:w2697, 9:w2696) -> (15:w2699:errorcluster)  [unwired: 2 in, 3 out]
                            n1426 = local write "data file error"(w2699) -> ()
                          }
                          frame #1 {
                            n1427 = Bundle(cluster=w2700, "STATUS"="T-RISE PASS") -> (w2702:T4)  [unwired: 2 in]
                            n1428 = local write "RESULT LAB03-2"(TRUE) -> ()
                            n1429 = local write "DISP LAB03-2"(w2702) -> ()
                          }
                        }
                      }
                      frame False {
                      }
                    }
                  }
                }
              }
              frame #6 {
                # "LAB04-1"
                n1430 = Equal?(x=w2705, y=2) -> (x = y?=w2708:bool)
                n1431 = local read "DISP LAB04-1"() -> (w2710:T4)
                n1432 = Unbundle(w2710) -> ("STATUS"=w2711:string)  [unwired: 2 out]
                n1433 = Equal?(x=w2711, y="RUN") -> (x = y?=w2707:bool)
                n1434 = And(x=w2707, y=w2708) -> (x .and. y?=w2706:bool)
                n1435 = case shown="True" w2706 {
                  tunnel: w2710 -> [_ w2714]
                  tunnel: w2704 -> [_ w2717]
                  frame False {
                  }
                  frame True {
                    n1436 = local read "SET LAB04-1"() -> (w2716:T5)
                    n1437 = local read "TDMS LAB04-1"() -> (w2713:refnum<k34>)
                    n1438 = Unbundle(w2714) -> ("CYCLE"=w2718:dbl)  [unwired: 2 out]
                    n1439 = Unbundle(w2716) -> ("T-RISE mins"=w2715:dbl)  [unwired: 4 out]
                    n1440 = Greater Or Equal?(x=w2718, y=w2717) -> (x >= y?=w2719:bool)
                    n1441 = case shown="True" w2719 {
                      tunnel: w2715 -> [w2722 _]
                      tunnel: w2714 -> [w2721 _]
                      tunnel: w2713 -> [w2720 _]
                      frame True {
                        n1442 = stacked-sequence {
                          tunnel: w2722 -> [w2725 _]
                          tunnel: w2721 -> [_ w2730]
                          tunnel: w2720 -> [w2723 _]
                          frame #0 {
                            n1443 = Build Array("T-RISE") -> (w2727:string[])
                            n1444 = Build Array(w2725) -> (w2726:dbl[])
                            n1445 = TDMS Write(0:w2723, 5:"TEST PASS", 7:w2727, 9:w2726) -> (15:w2729:errorcluster)  [unwired: 2 in, 3 out]
                            n1446 = local write "data file error"(w2729) -> ()
                          }
                          frame #1 {
                            n1447 = Bundle(cluster=w2730, "STATUS"="T-RISE PASS") -> (w2732:T4)  [unwired: 2 in]
                            n1448 = local write "RESULT LAB04-1"(TRUE) -> ()
                            n1449 = local write "DISP LAB04-1"(w2732) -> ()
                          }
                        }
                      }
                      frame False {
                      }
                    }
                  }
                }
              }
              frame #7 {
                # "LAB04-2"
                n1450 = Equal?(x=w2735, y=2) -> (x = y?=w2738:bool)
                n1451 = local read "DISP LAB04-2"() -> (w2740:T4)
                n1452 = Unbundle(w2740) -> ("STATUS"=w2741:string)  [unwired: 2 out]
                n1453 = Equal?(x=w2741, y="RUN") -> (x = y?=w2737:bool)
                n1454 = And(x=w2737, y=w2738) -> (x .and. y?=w2736:bool)
                n1455 = case shown="True" w2736 {
                  tunnel: w2740 -> [_ w2744]
                  tunnel: w2734 -> [_ w2747]
                  frame False {
                  }
                  frame True {
                    n1456 = local read "SET LAB04-2"() -> (w2746:T5)
                    n1457 = local read "TDMS LAB04-2"() -> (w2743:refnum<k34>)
                    n1458 = Unbundle(w2744) -> ("CYCLE"=w2748:dbl)  [unwired: 2 out]
                    n1459 = Unbundle(w2746) -> ("T-RISE mins"=w2745:dbl)  [unwired: 4 out]
                    n1460 = Greater Or Equal?(x=w2748, y=w2747) -> (x >= y?=w2749:bool)
                    n1461 = case shown="True" w2749 {
                      tunnel: w2745 -> [w2752 _]
                      tunnel: w2744 -> [w2751 _]
                      tunnel: w2743 -> [w2750 _]
                      frame True {
                        n1462 = stacked-sequence {
                          tunnel: w2752 -> [w2755 _]
                          tunnel: w2751 -> [_ w2760]
                          tunnel: w2750 -> [w2753 _]
                          frame #0 {
                            n1463 = Build Array("T-RISE") -> (w2757:string[])
                            n1464 = Build Array(w2755) -> (w2756:dbl[])
                            n1465 = TDMS Write(0:w2753, 5:"TEST PASS", 7:w2757, 9:w2756) -> (15:w2759:errorcluster)  [unwired: 2 in, 3 out]
                            n1466 = local write "data file error"(w2759) -> ()
                          }
                          frame #1 {
                            n1467 = Bundle(cluster=w2760, "STATUS"="T-RISE PASS") -> (w2762:T4)  [unwired: 2 in]
                            n1468 = local write "RESULT LAB04-2"(TRUE) -> ()
                            n1469 = local write "DISP LAB04-2"(w2762) -> ()
                          }
                        }
                      }
                      frame False {
                      }
                    }
                  }
                }
              }
              frame #8 {
                # "LAB05-1"
                n1470 = Equal?(x=w2765, y=2) -> (x = y?=w2768:bool)
                n1471 = local read "DISP LAB05-1"() -> (w2770:T4)
                n1472 = Unbundle(w2770) -> ("STATUS"=w2771:string)  [unwired: 2 out]
                n1473 = Equal?(x=w2771, y="RUN") -> (x = y?=w2767:bool)
                n1474 = And(x=w2767, y=w2768) -> (x .and. y?=w2766:bool)
                n1475 = case shown="True" w2766 {
                  tunnel: w2770 -> [_ w2774]
                  tunnel: w2764 -> [_ w2777]
                  frame False {
                  }
                  frame True {
                    n1476 = local read "SET LAB05-1"() -> (w2776:T5)
                    n1477 = local read "TDMS LAB05-1"() -> (w2773:refnum<k34>)
                    n1478 = Unbundle(w2774) -> ("CYCLE"=w2778:dbl)  [unwired: 2 out]
                    n1479 = Unbundle(w2776) -> ("T-RISE mins"=w2775:dbl)  [unwired: 4 out]
                    n1480 = Greater Or Equal?(x=w2778, y=w2777) -> (x >= y?=w2779:bool)
                    n1481 = case shown="True" w2779 {
                      tunnel: w2775 -> [w2782 _]
                      tunnel: w2774 -> [w2781 _]
                      tunnel: w2773 -> [w2780 _]
                      frame True {
                        n1482 = stacked-sequence {
                          tunnel: w2782 -> [w2785 _]
                          tunnel: w2781 -> [_ w2790]
                          tunnel: w2780 -> [w2783 _]
                          frame #0 {
                            n1483 = Build Array("T-RISE") -> (w2787:string[])
                            n1484 = Build Array(w2785) -> (w2786:dbl[])
                            n1485 = TDMS Write(0:w2783, 5:"TEST PASS", 7:w2787, 9:w2786) -> (15:w2789:errorcluster)  [unwired: 2 in, 3 out]
